vi "Command_Turret_MoveToPosition.vi"(7 "Startup":bool, 9 "Timeout":dbl=5000.0, 10 "Speed":dbl=1.0, 11 "Goal_Position":dbl=-16700.0) -> (2 "Turret_Speed":dbl=-1.0, 4 "Reint":bool, 6 "Completed":bool)   [LabVIEW 2019]
uses:
  Command_Execution_State.ctl
  Globals/Sensor_Values.vi
panel:
  in  "Acceptable_Error":dbl
  in  "Kp":dbl=0.001
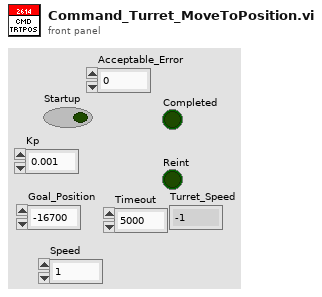
[diagram p1: front panel]
types:
  T1 = typedef "Command_Execution_State.ctl" = enum16{"Initialize", "Execute", "Finish"}
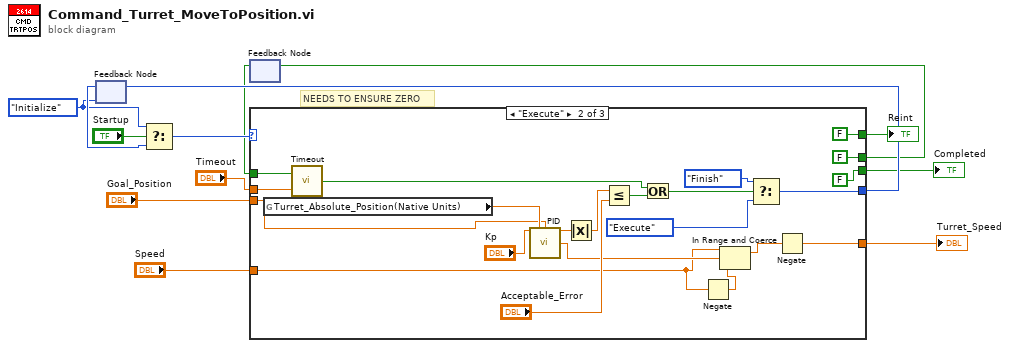
[diagram p0: block diagram]
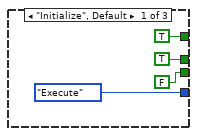
[diagram p2: hidden frame]
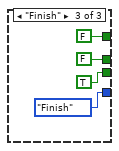
[diagram p3: hidden frame]
diagram:
  w7 = Command_Execution_State."Initialize" ("Play State")
  # "NEEDS TO ENSURE ZERO"
  n1 = feedback #1(w7) -> (w11:T1)
  n2 = Select(t=w7, s="Startup", f=w11) -> (s? t:f=w13:T1)
  n3 = feedback #2() -> (w4:bool)  [unwired: 1 in]
  n4 = case shown="\"Execute\"" w13 {
    tunnel: [Command_Execution_State."Execute" ("Play State") w30 Command_Execution_State."Finish" ("Play State")] -> w12
    tunnel: [FALSE FALSE TRUE] -> w10
    tunnel: [TRUE FALSE FALSE] -> w8
    tunnel: "Goal_Position" -> [_ w36 _]
    tunnel: w4 -> [_ w34 _]
    tunnel: [TRUE FALSE FALSE] -> w5
    tunnel: "Timeout" -> [_ w32 _]
    tunnel: [_ w18 _] -> w2
    tunnel: "Speed" -> [_ w20 _]
    frame "Initialize", Default {
    }
    frame "Execute" {
      n5 = global read "Sensor_Values.vi" "Turret_Absolute_Position(Native Units)"() -> (w37:dbl)
      n6 = call "Timeout.vi"("Timeout"=w32, "Initialize"=w34) -> ("Timed Out?"=w28:bool)
      n7 = call "PID.vi"("Kp"="Kp", "Process Variable"=w37, "Goal"=w36) -> ("Current Error"=w27:dbl, "Command"=w22:dbl)  [unwired: 10 in, 1 out]
      n8 = Absolute Value(x=w27) -> (abs(x)=w25:dbl)
      n9 = Less Or Equal?(x=w25, y="Acceptable_Error") -> (x <= y?=w26:bool)
      n10 = Or(x=w28, y=w26) -> (x .or. y?=w23:bool)
      n11 = Negate(x=w20) -> (-x=w21:dbl)
      n12 = In Range and Coerce(upper limit=w20, x=w22, lower limit=w21) -> (coerced(x)=w19:dbl)  [unwired: 1 out]
      n13 = Select(t=Command_Execution_State."Finish" ("Play State"), s=w23, f=Command_Execution_State."Execute" ("Play State")) -> (s? t:f=w30:T1)
      n14 = Negate(x=w19) -> (-x=w18:dbl)
    }
    frame "Finish" {
    }
  }
  "Completed" <- w10
  "Reint" <- w8
  "Turret_Speed" <- w2
  n15 = feedback-in #1(w12) -> ()
  n16 = feedback-in #2(w5) -> ()
